vi "Apply Changes.vi"(8 "error in (no error)":errorcluster, 11 "New Project Wizard in":refnum<class "New Project Wizard.lvclass">) -> (0 "error out":errorcluster, 3 "New Project Wizard out":refnum<class "New Project Wizard.lvclass">)   [LabVIEW 2013, in "SET Project Editor.lvlib" / "New Project Wizard.lvclass"]
uses:
  New Project Wizard.lvclass
  UI Wizard/UI Wizard.lvclass
  <vilib>/ActorFramework/Actor/Actor.lvclass/Actor.ctl
  UI Wizard/UI Wizard.lvclass/UI Wizard.ctl
  New Project Wizard.lvclass/New Project Wizard.ctl
  <vilib>/ActorFramework/Message Enqueuer/Message Enqueuer.lvclass/Message Enqueuer.ctl
  UI Wizard/Read Project Data ref.vi
  <vilib>/ActorFramework/Message Enqueuer/Enqueue.vi
  <vilib>/ActorFramework/Message Priority Queue/Priority Enqueue.vi
  Controller Messages/Set Modified Flag Msg/Set Modified Flag Msg.lvclass
  Controller Messages/UI Refresh Msg/UI Refresh Msg.lvclass
  <vilib>/ActorFramework/Actor/Actor.lvclass
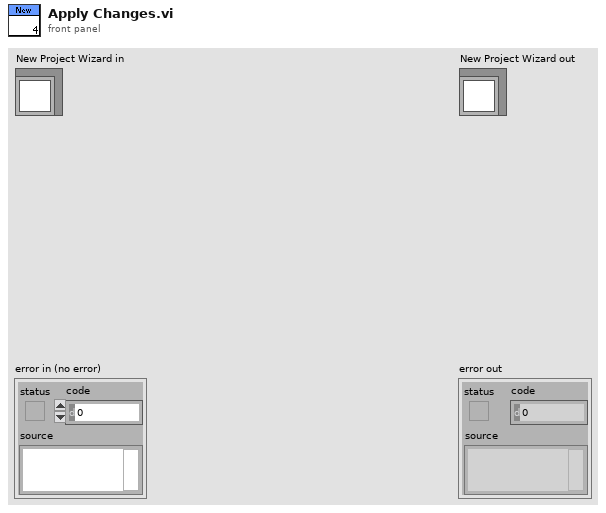
[diagram p1: front panel]
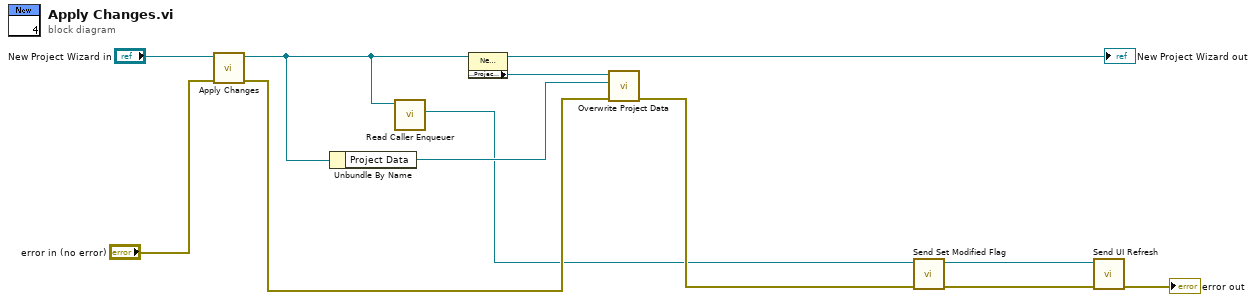
[diagram p0: block diagram]
diagram:
  n1 = call-parent "Apply Changes.vi"("error in (no error)"="error in (no error)", "UI Wizard in"="New Project Wizard in") -> ("error out"=w5:errorcluster, "UI Wizard out"=w10:refnum<class "New Project Wizard.lvclass">)  [unwired: 8 in]
  n2 = Unbundle By Name(w10) -> ("Project Data"=w6:refnum<class "Project Data.lvclass">)
  n3 = call <vilib>:"Read Caller Enqueuer.vi"("Actor"=w10) -> ("Caller Enqueuer"=w2:refnum<class "Message Enqueuer.lvclass">)  [unwired: 10 in]
  n4 = property class="New Project Wizard.lvclass"(reference=w10) -> (reference out=→"New Project Wizard out":refnum<class "New Project Wizard.lvclass">, "Properties:Project Data ref"=w7:refnum<data-value>)  [unwired: 1 in, 1 out]
  n5 = call "Overwrite Project Data.vi"("error in (no error)"=w5, "Project Data"=w6, "Project Data ref in"=w7) -> ("error out"=w3:errorcluster)  [unwired: 7 in, 1 out]
  n6 = call "Send Set Modified Flag.vi"("error in (no error)"=w3, "Message Enqueuer"=w2) -> ("error out"=w4:errorcluster, "Message Enqueuer out"=w1:refnum<class "Message Enqueuer.lvclass">)  [unwired: 8 in]
  n7 = call "Send UI Refresh.vi"("error in (no error)"=w4, "Message Enqueuer"=w1) -> ("error out"=→"error out":errorcluster)  [unwired: 8 in, 1 out]
